vi "Lab 6 II.vi"() -> ()   [LabVIEW 2021]
panel:
  in  "Table Control":string[][](table)
  out "?":bool
  in  "Password:":string
  in  "Username:":string
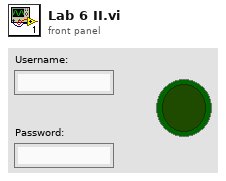
[diagram p1: front panel]
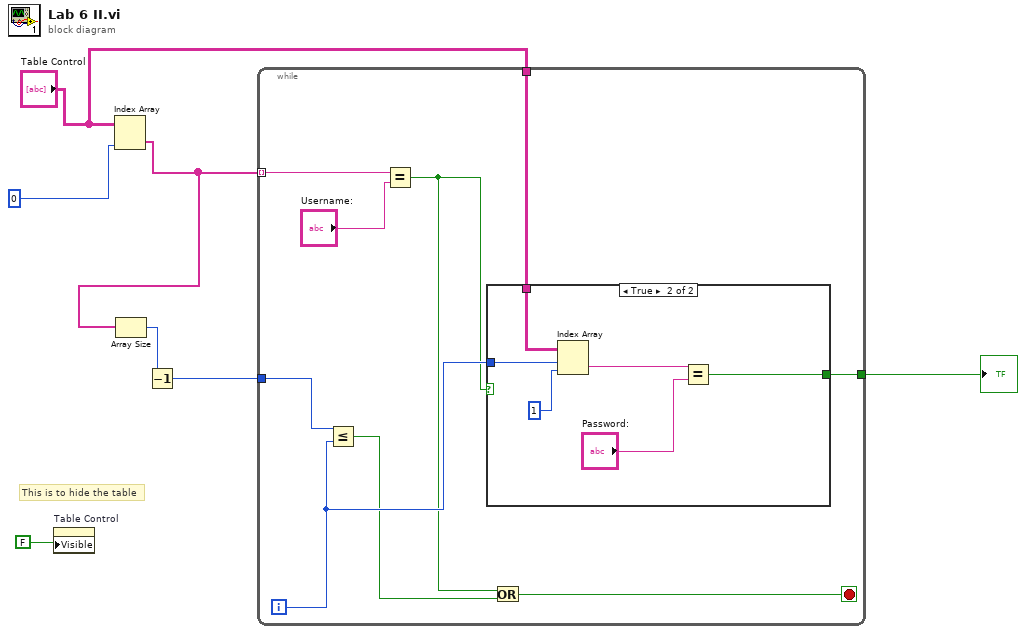
[diagram p0: block diagram]
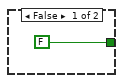
[diagram p2: hidden frame]
diagram:
  # "This is to hide the table"
  n1 = property on="Table Control" class="Tbl (strict)"("Visible"=FALSE) -> ()  [unwired: 2 in, 2 out]
  n2 = Index Array "Index Array"(array="Table Control", index (col)=0) -> (element=w4:string[])  [unwired: 1 in]
  n3 = Array Size(array=w4) -> (size(s)=w3:i32)
  n4 = Decrement(x=w3) -> (x-1=w2:i32)
  n5 = while {
    tunnel: w4 -> [w16] mode=indexing
    tunnel: "Table Control" -> [w14]
    tunnel: [w13] -> w5
    tunnel: w2 -> [w12]
    i -> [w11]
    stop <- w8 stop-if-true
    n6 = Less Or Equal?(x=w12, y=w11) -> (x <= y?=w9:bool)
    n7 = Equal?(x=w16, y="Username:") -> (x = y?=w10:bool)
    n8 = case shown="True" w10 {
      tunnel: w14 -> [_ w23]
      tunnel: [FALSE w19] -> w13
      tunnel: w11 -> [_ w18]
      frame False {
      }
      frame True {
        n9 = Index Array(array=w23, index (row)=w18, index (col)=1) -> (element=w21:string)
        n10 = Equal?(x=w21, y="Password:") -> (x = y?=w19:bool)
      }
    }
    n11 = Or(x=w10, y=w9) -> (x .or. y?=w8:bool)
  }
  "?" <- w5
